vi "Sub_timing calc.vi"(0 "Experiment In":T1) -> (1 "Experimental Results OUT":T2={"time_average_cycle"=0.0, "measured_frequency"=[], "date_time"="", "estimated_pin_node"=[], "time_cycle_start"=[], "measured_pin_location"=[], "estimated_frequency"=[], "acceleration_data"=[], "accelerometer_sample_rate"=0.0, "displacement_sample_rate"=0.0, "time_compare_start"=array[564 elements], "time_subsample_start"=array[564 elements], "time_FEA_start"=array[564 elements], "time_FEA_end"=array[564 elements], "time_cycle_end"=array[564 elements], "time_accelerometer_aquire_start"=array[564 elements], "time_frequency_calculations_start"=array[564 elements], "time_frequency_calculations_end"=array[564 elements], "measured_pin_location_tt"=array[564 elements], "time_ACC_data_collection_start"=0.0, "time_acceleration_data"=array[564 elements], "estimated_pin_location"=array[564 elements], "scaling_factor_Hz_per_pin_to_frequency_resolution"=1.0, "Std_Dev_equale_particles_divided_3"=TRUE, "Auto_FFT_length"=TRUE, "windowed_acc_data"=array1x564[564 elements], "FFT"=array1x564[564 elements]}, 2 "mean":dbl format="%0.10f")   [LabVIEW 2021]
uses:
  <vilib>/Analysis/baseanly.llb/Mean (DBL).vi
  <vilib>/Analysis/NI_AALBase.lvlib
panel:
  out "number of iterations run":i32
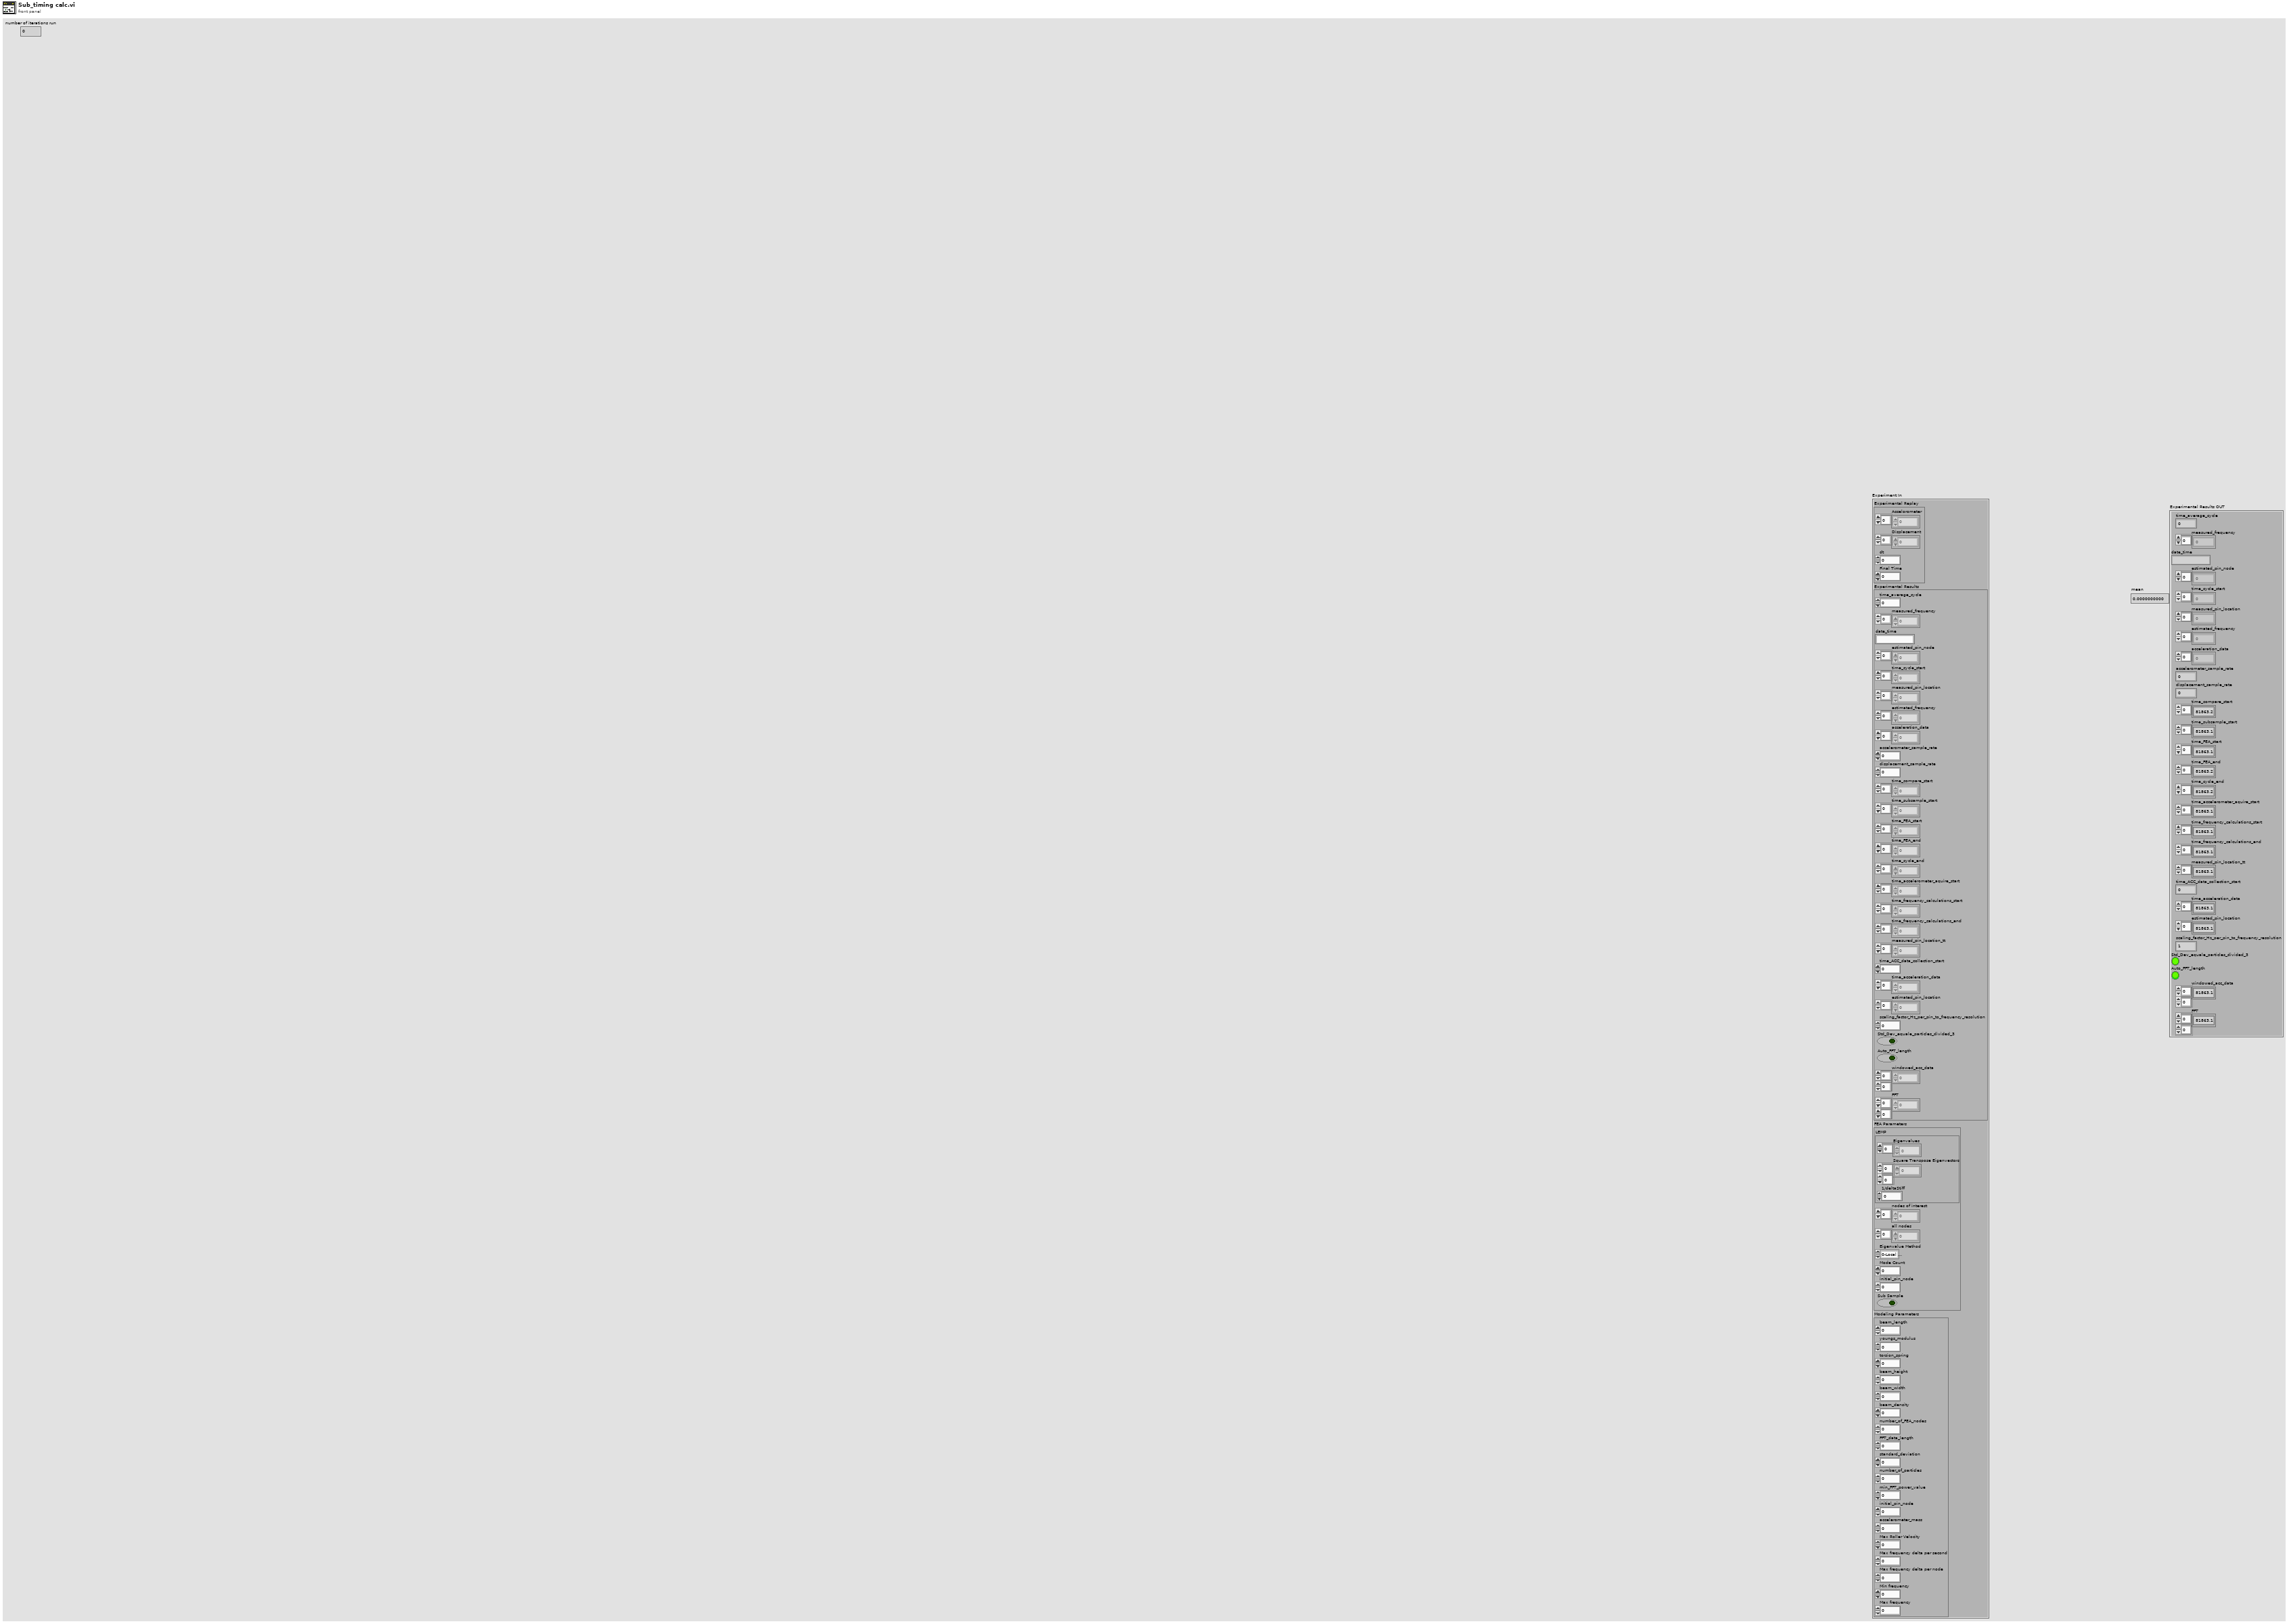
[diagram p1: front panel]
types:
  T1 = cluster{"Experimental Replay":cluster{"Accelorometer":dbl[], "Displacement":dbl[], "dt":dbl, "Final Time":dbl}, "Experimental Results":cluster{"time_average_cycle":dbl, "measured_frequency":dbl[], "date_time":string, "estimated_pin_node":i32[], "time_cycle_start":dbl[], "measured_pin_location":dbl[], "estimated_frequency":dbl[], "acceleration_data":dbl[], "accelerometer_sample_rate":dbl, "displacement_sample_rate":dbl, "time_compare_start":dbl[], "time_subsample_start":dbl[], "time_FEA_start":dbl[], "time_FEA_end":dbl[], "time_cycle_end":dbl[], "time_accelerometer_aquire_start":dbl[], "time_frequency_calculations_start":dbl[], "time_frequency_calculations_end":dbl[], "measured_pin_location_tt":dbl[], "time_ACC_data_collection_start":dbl, "time_acceleration_data":dbl[], "estimated_pin_location":dbl[], "scaling_factor_Hz_per_pin_to_frequency_resolution":dbl, "Std_Dev_equale_particles_divided_3":bool, "Auto_FFT_length":bool, "windowed_acc_data":dbl[][], "FFT":dbl[][]}, "FEA Parameters":cluster{"LEMP":cluster{"Eigenvalues":dbl[], "Square Transpose Eigenvectors":dbl[][], "1/deltaStiff":dbl}, "nodes of interest":i32[], "all nodes":i32[], "Eigenvalue Method":enum16{"0-Local Eigen Modification Procedure", "1-LabVIEW generalized eigenvalues", "2-LabVIEW M^-1K eigenvalues", "3-LabVIEW Cholesky Factorization", "4-Cholesky Factorization CPU SGL", "5-Cholesky Factorization CPU FXP", "6-Cholesky Factorization FPGA SGL", "7-Cholesky Factorization FPGA SGL SCL"}, "Mode Count":i32, "initial_pin_node":i32, "Sub Sample":bool}, "Modeling Parameters":cluster{"beam_length":dbl, "youngs_modulus":dbl, "torsion_spring":dbl, "beam_height":dbl, "beam_width":dbl, "beam_density":dbl, "number_of_FEA_nodes":i32, "FFT_data_length":i32, "standard_deviation":dbl, "number_of_particles":i32, "min_FFT_power_value":dbl, "initial_pin_node":i32, "accelerometer_mass":dbl, "Max Roller Velocity":dbl, "Max frequency delta per second":dbl, "Max frequency delta per node":dbl, "Min frequency":dbl, "Max frequency":dbl}}
  T2 = cluster{"time_average_cycle":dbl, "measured_frequency":dbl[], "date_time":string, "estimated_pin_node":i32[], "time_cycle_start":dbl[], "measured_pin_location":dbl[], "estimated_frequency":dbl[], "acceleration_data":dbl[], "accelerometer_sample_rate":dbl, "displacement_sample_rate":dbl, "time_compare_start":dbl[], "time_subsample_start":dbl[], "time_FEA_start":dbl[], "time_FEA_end":dbl[], "time_cycle_end":dbl[], "time_accelerometer_aquire_start":dbl[], "time_frequency_calculations_start":dbl[], "time_frequency_calculations_end":dbl[], "measured_pin_location_tt":dbl[], "time_ACC_data_collection_start":dbl, "time_acceleration_data":dbl[], "estimated_pin_location":dbl[], "scaling_factor_Hz_per_pin_to_frequency_resolution":dbl, "Std_Dev_equale_particles_divided_3":bool, "Auto_FFT_length":bool, "windowed_acc_data":dbl[][], "FFT":dbl[][]}
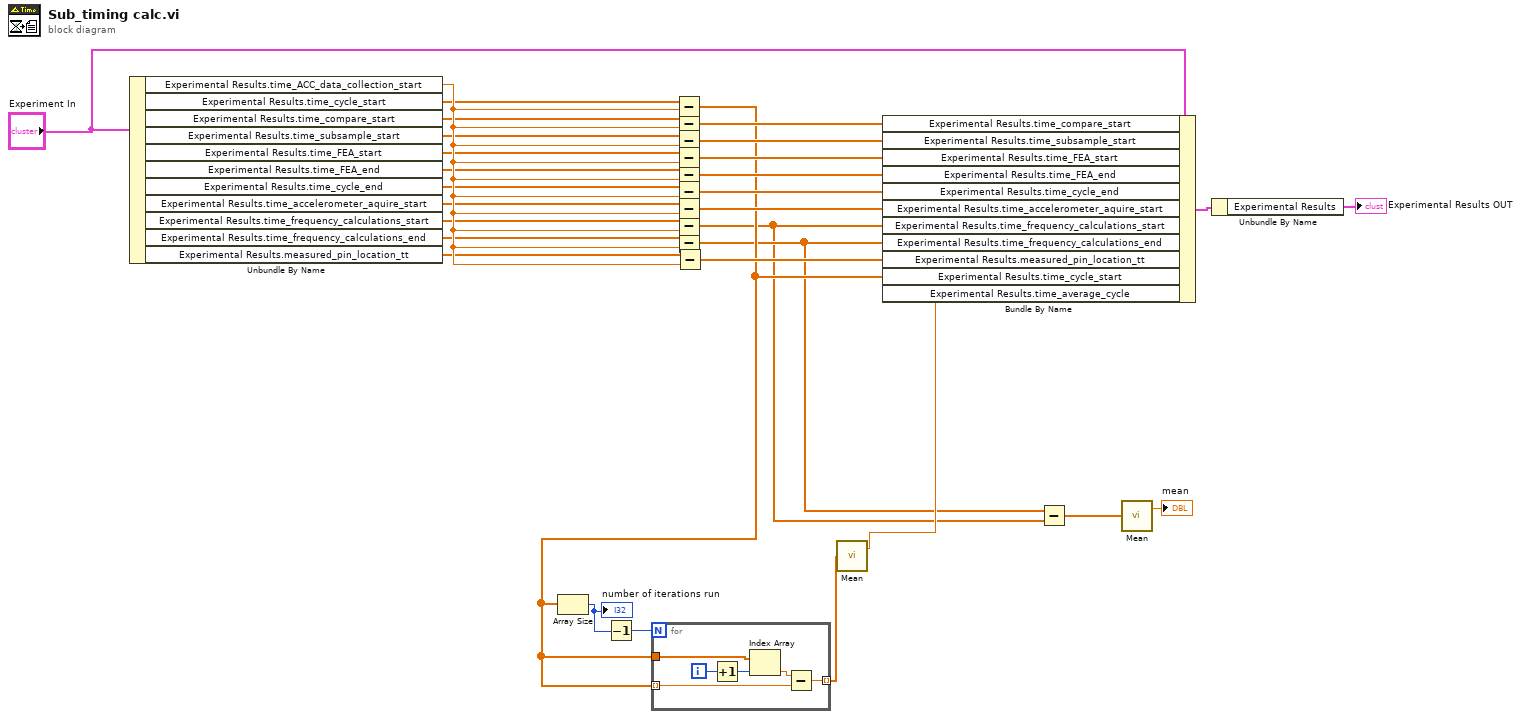
[diagram p0: block diagram]
diagram:
  n1 = Unbundle By Name("Experiment In") -> ("Experimental Results.time_ACC_data_collection_start"=w11:dbl, "Experimental Results.time_cycle_start"=w10:dbl[], "Experimental Results.time_compare_start"=w9:dbl[], "Experimental Results.time_subsample_start"=w8:dbl[], "Experimental Results.time_FEA_start"=w7:dbl[], "Experimental Results.time_FEA_end"=w6:dbl[], "Experimental Results.time_cycle_end"=w5:dbl[], "Experimental Results.time_accelerometer_aquire_start"=w1:dbl[], "Experimental Results.time_frequency_calculations_start"=w2:dbl[], "Experimental Results.time_frequency_calculations_end"=w3:dbl[], "Experimental Results.measured_pin_location_tt"=w4:dbl[])
  n2 = Subtract(x=w10, y=w11) -> (x-y=w19:dbl[])
  n3 = Array Size(array=w19) -> (size(s)=w22:i32)
  "number of iterations run" <- w22
  n4 = Decrement(x=w22) -> (x-1=w23:i32)
  n5 = for {
    N: w23 -> [_]
    tunnel: w19 -> [w36] mode=indexing
    tunnel: w19 -> [w35]
    tunnel: [w31] -> w21 mode=indexing
    i -> [w34]
    n6 = Increment(x=w34) -> (x+1=w33:i32)
    n7 = Index Array(array=w35, index=w33) -> (element=w32:dbl)
    n8 = Subtract(x=w32, y=w36) -> (x-y=w31:dbl)
  }
  n9 = Subtract(x=w9, y=w11) -> (x-y=w30:dbl[])
  n10 = Subtract(x=w8, y=w11) -> (x-y=w29:dbl[])
  n11 = Subtract(x=w7, y=w11) -> (x-y=w28:dbl[])
  n12 = Subtract(x=w6, y=w11) -> (x-y=w24:dbl[])
  n13 = Subtract(x=w5, y=w11) -> (x-y=w27:dbl[])
  n14 = Subtract(x=w1, y=w11) -> (x-y=w26:dbl[])
  n15 = Subtract(x=w2, y=w11) -> (x-y=w17:dbl[])
  n16 = Subtract(x=w3, y=w11) -> (x-y=w18:dbl[])
  n17 = Subtract(x=w4, y=w11) -> (x-y=w25:dbl[])
  n18 = call-poly <vilib>:"Mean.vi"("X"=w21) -> ("mean"=w20:dbl)  [unwired: 1 out]
  n19 = Bundle By Name(cluster="Experiment In", "Experimental Results.time_compare_start"=w30, "Experimental Results.time_subsample_start"=w29, "Experimental Results.time_FEA_start"=w28, "Experimental Results.time_FEA_end"=w24, "Experimental Results.time_cycle_end"=w27, "Experimental Results.time_accelerometer_aquire_start"=w26, "Experimental Results.time_frequency_calculations_start"=w17, "Experimental Results.time_frequency_calculations_end"=w18, "Experimental Results.measured_pin_location_tt"=w25, "Experimental Results.time_cycle_start"=w19, "Experimental Results.time_average_cycle"=w20) -> (w13:T1)
  n20 = Subtract(x=w18, y=w17) -> (x-y=w16:dbl[])
  n21 = call-poly <vilib>:"Mean.vi"("X"=w16) -> ("mean"=→"mean":dbl)  [unwired: 1 out]
  n22 = Unbundle By Name(w13) -> ("Experimental Results"=→"Experimental Results OUT":T2)
